vi "HR_Calculate_Percentage.vi"(8 "error in (no error)":errorcluster, 11 "HR Data Structure in":T3) -> (0 "error out":errorcluster, 2 "reversed array":dbl[](array[numeric]), 3 "output cluster":T2)   [LabVIEW 2021]
uses:
  HR Data Structure.ctl
  Runner's Data.ctl
  Raw Data.ctl
  e6a1e60f-9a01-4349-afc9-f9c02ba13944.vi
  <vilib>/Comparison/Less/Less Functor/Less Functor.lvclass
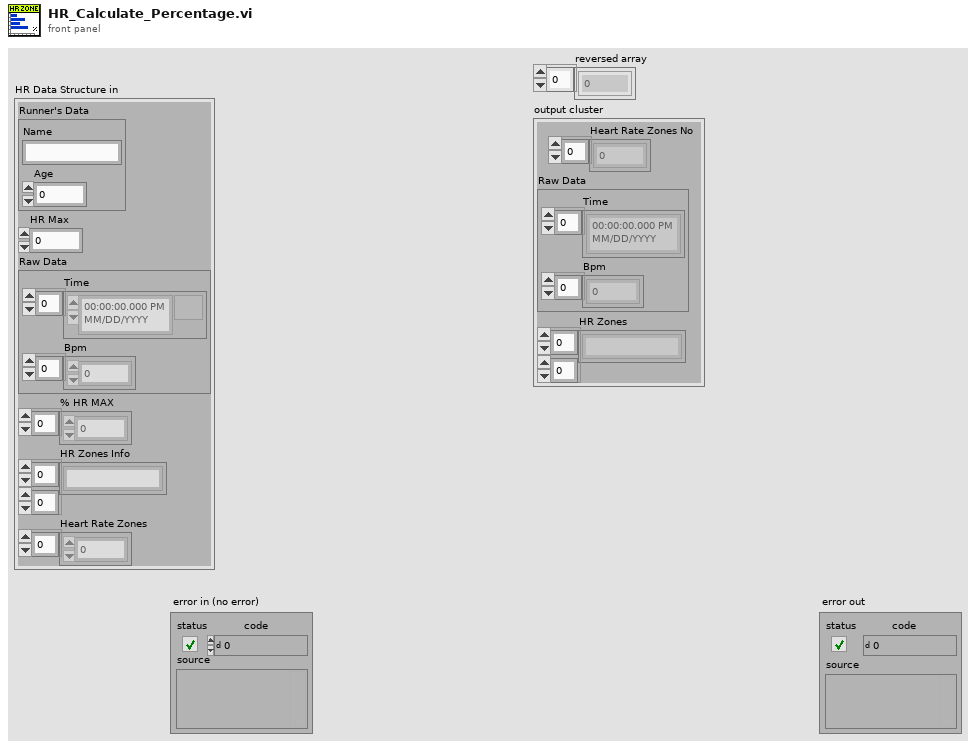
[diagram p1: front panel]
types:
  T1 = typedef "Raw Data.ctl" = cluster{"Time":timestamp[], "Bpm":i32[]}
  T2 = cluster{"Heart Rate Zones No":dbl[], "Raw Data":T1, "HR Zones":string[][]}
  T3 = typedef "HR Data Structure.ctl" = cluster{"Runner's Data":T4, "HR Max":i32, "Raw Data":T1, "% HR MAX ":dbl[], "HR Zones Info":string[][], "Heart Rate Zones":dbl[]}
  T4 = typedef "Runner's Data.ctl" = cluster{"Name":string, "Age":i32}
  T5 = cluster{i32[], "Raw Data":T1, "HR Zones Info":string[][]}
  T6 = cluster{"Heart Rate Zones":dbl[], "Raw Data":T1, "HR Zones Info":string[][]}
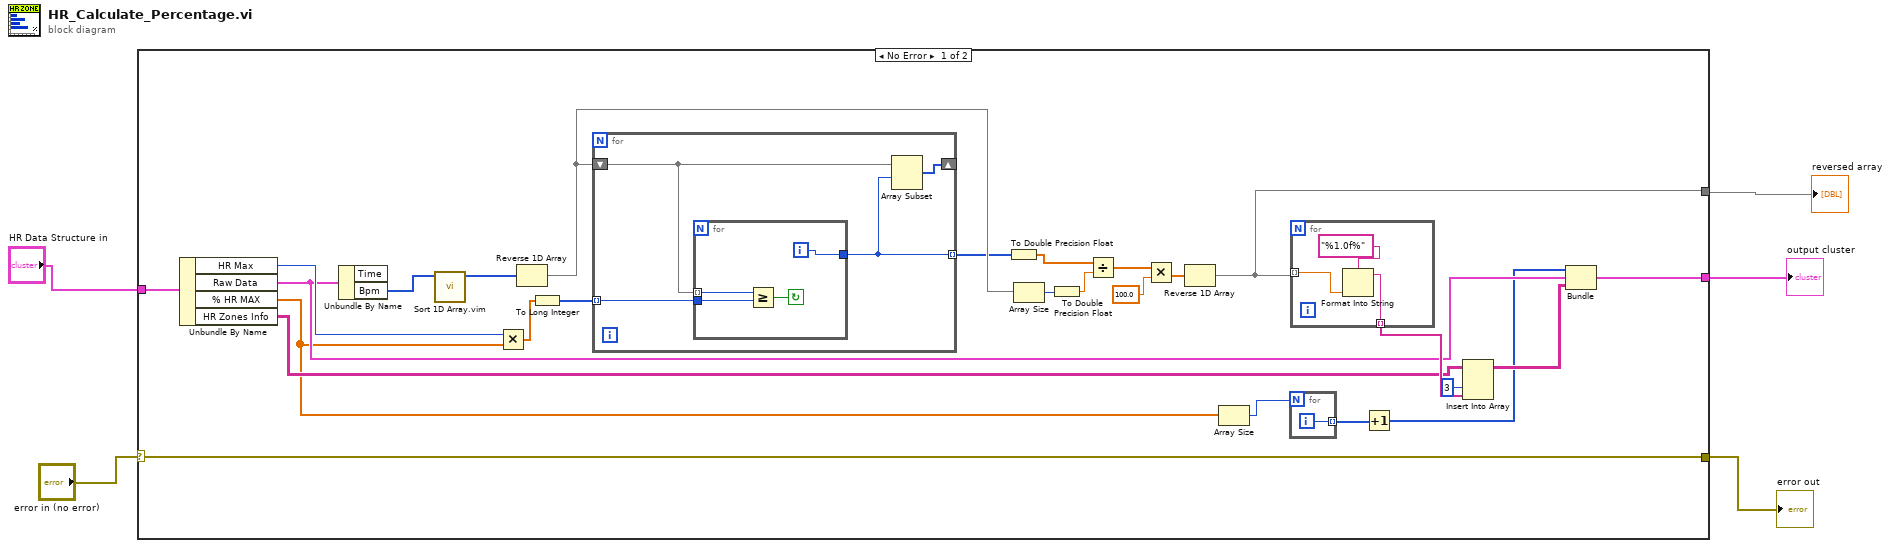
[diagram p0: block diagram]
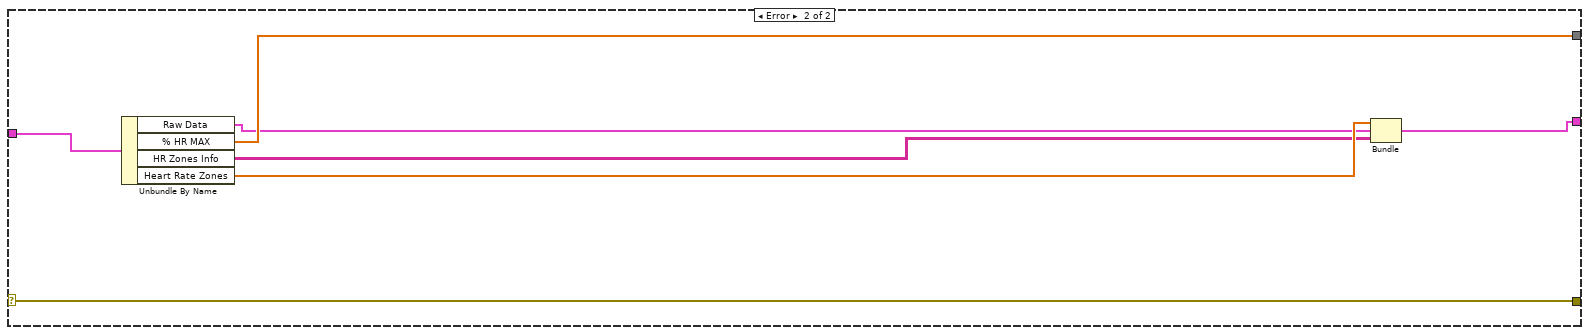
[diagram p2: hidden frame]
diagram:
  n1 = case shown="No Error" "error in (no error)" {
    selector: "error in (no error)" -> [w18 w50]
    tunnel: "HR Data Structure in" -> [w15 w49]
    tunnel: [w18 w50] -> w3
    tunnel: [w14 w48] -> w2
    tunnel: [w6 w47] -> w1
    frame No Error {
      n2 = Unbundle By Name(w15) -> ("HR Max"=w30:i32, "Raw Data"=w13:T1, "% HR MAX"=w10:dbl[], "HR Zones Info"=w16:string[][])
      n3 = Unbundle By Name(w13) -> ("Bpm"=w29:i32[])  [unwired: 1 out]
      n4 = call "Sort 1D Array.vim"("unsorted array"=w29) -> ("sorted array"=w19:i32[])  [unwired: 10 in]
      n5 = Multiply(x=w30, y=w10) -> (x*y=w31:dbl[])
      n6 = Reverse 1D Array(array=w19) -> (reversed array=w21:i32[])
      n7 = To Long Integer(number=w31) -> (32bit integer=w28:i32[])
      n8 = for {
        shift-right: [w38] -> _
        shift-left: w21 -> [w39]
        tunnel: [w37] -> w20 mode=indexing
        tunnel: w28 -> [w36] mode=indexing
        n9 = for {
          tunnel: w39 -> [w40] mode=indexing
          tunnel: [w43] -> w37
          tunnel: w36 -> [w41]
          i -> [w43]
          stop <- w42 continue-if-true
          n10 = Greater Or Equal?(x=w40, y=w41) -> (x >= y?=w42:bool)
        }
        n11 = Array Subset(array=w39, index=w37) -> (w38:i32[])  [unwired: 1 in]
      }
      n12 = To Double Precision Float(number=w20) -> (double precision float=w24:dbl[])
      n13 = Array Size(array=w21) -> (size(s)=w22:i32)
      n14 = To Double Precision Float(number=w22) -> (double precision float=w23:dbl)
      n15 = Divide(x=w24, y=w23) -> (x/y=w26:dbl[])
      n16 = Multiply(x=w26, y=100.0) -> (x*y=w27:dbl[])
      n17 = Reverse 1D Array(array=w27) -> (reversed array=w14:dbl[])
      n18 = Array Size(array=w10) -> (size(s)=w9:i32)
      n19 = for {
        N: w9 -> [_]
        tunnel: [w32] -> w8 mode=indexing
        i -> [w32]
      }
      n20 = for {
        tunnel: w14 -> [w34] mode=indexing
        tunnel: [w33] -> w17 mode=indexing
        n21 = Format Into String(format string="%1.0f%", w34) -> (resulting string=w33:string)  [unwired: 2 in, 1 out]
      }
      n22 = Increment(x=w8) -> (x+1=w7:i32[])
      n23 = Insert Into Array(array=w16, index (col)=3 ("disabled index (col)"), new element=w17) -> (w12:string[][])  [unwired: 1 in]
      n24 = Bundle(w7, "Raw Data"=w13, "HR Zones Info"=w12) -> (w6:T5)  [unwired: 1 in]
    }
    frame Error {
      n25 = Unbundle By Name(w49) -> ("Raw Data"=w45:T1, "% HR MAX"=w48:dbl[], "HR Zones Info"=w44:string[][], "Heart Rate Zones"=w46:dbl[])
      n26 = Bundle("Heart Rate Zones"=w46, "Raw Data"=w45, "HR Zones Info"=w44) -> (w47:T6)  [unwired: 1 in]
    }
  }
  "error out" <- w3
  "reversed array" <- w2
  "output cluster" <- w1
